vi "adam-4069-basic.vi"() -> ()   [LabVIEW 2024]
uses:
  <vilib>/Instr/_visa.llb/VISA Configure Serial Port (Instr).vi
panel:
  out "Stop Pressed":bool
  out "On Pressed":bool
  out "return count":u32
  out "read buffer":string
  out "error out":errorcluster
  out "return count":u32
  in  "Stop Program":bool
  in  "Off":bool
  in  "On":bool
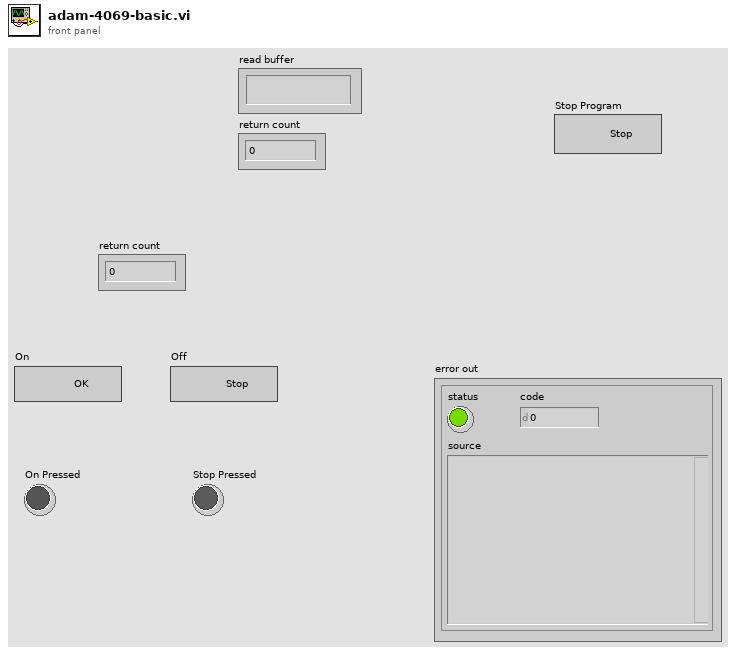
[diagram p1: front panel]
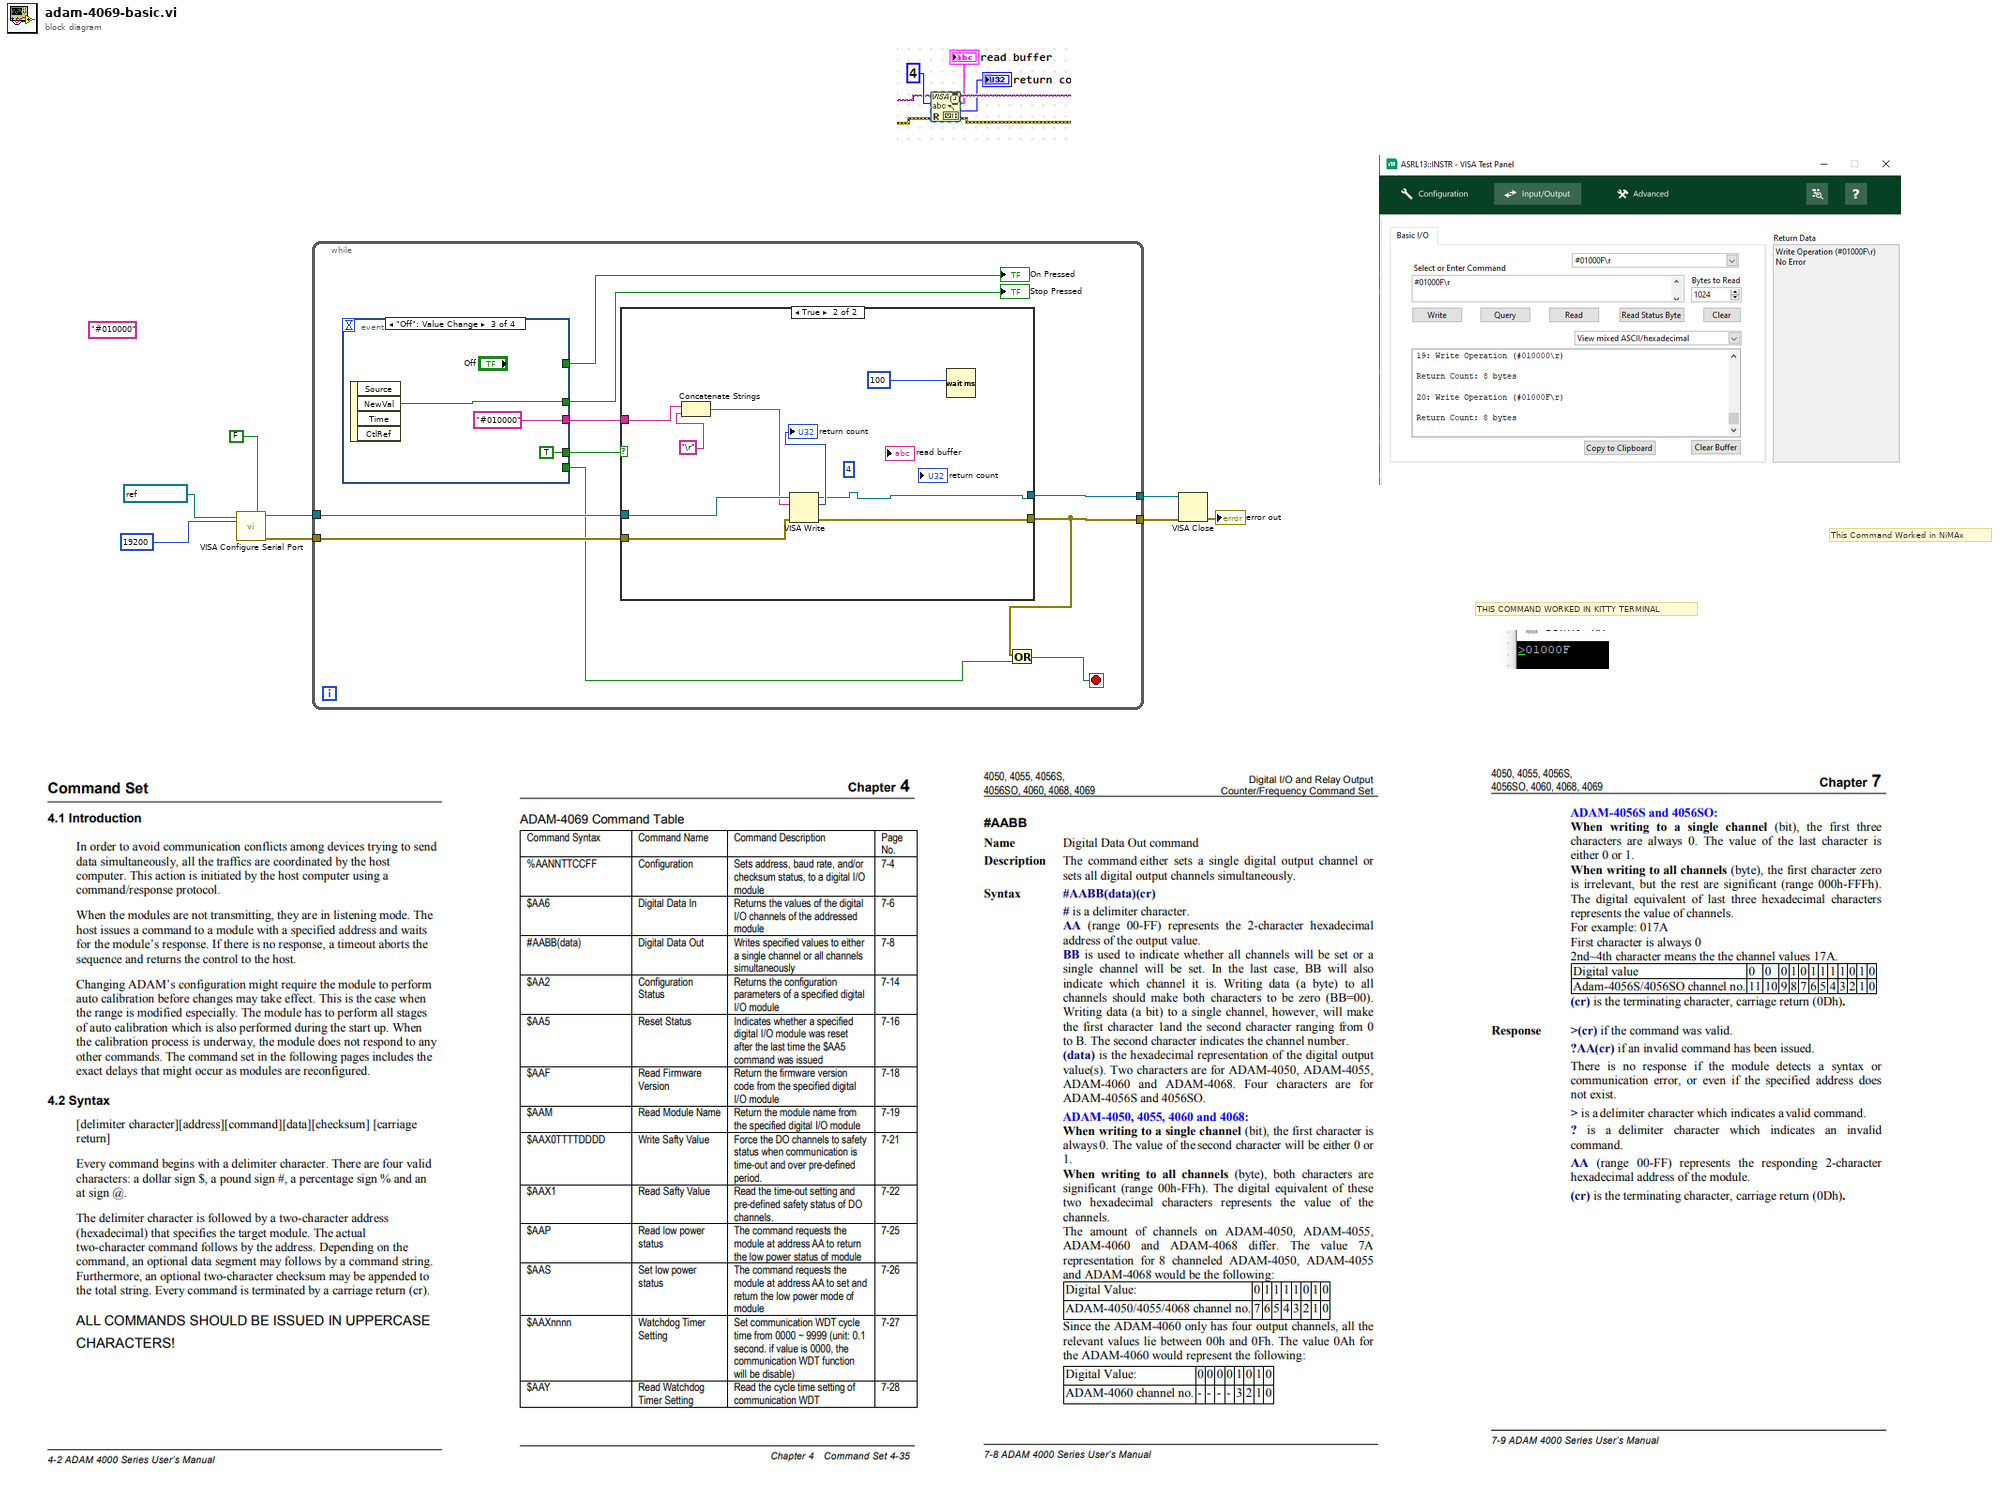
[diagram p0: block diagram]
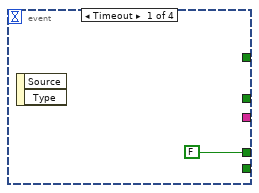
[diagram p2: hidden frame]
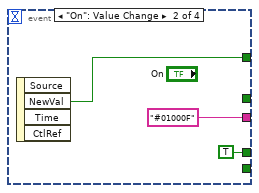
[diagram p3: hidden frame]
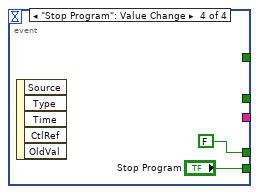
[diagram p4: hidden frame]
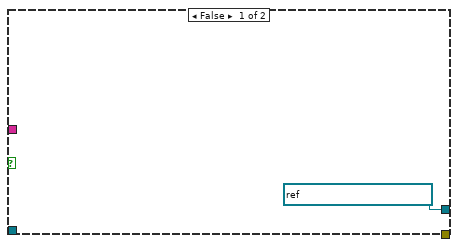
[diagram p5: hidden frame]
diagram:
  (unwired) "#010000" ("write buffer")
  # "This Command Worked in NiMAx"
  # "THIS COMMAND WORKED IN KITTY TERMINAL"
  n1 = call-poly "VISA Configure Serial Port"("VISA resource name"=refnum<visa-resource-name> "COM10", "Enable Termination\nChar (T)"=FALSE ("Enable Termination\nChar (T)"), "baud rate (9600)"=u32 19200) -> ("VISA resource name out"=w3:refnum<visa-resource-name>, "error out"=w2:errorcluster)  [unwired: 11 in]
  n2 = while {
    tunnel: [w18] -> w8
    tunnel: [w9] -> w7
    tunnel: w3 -> [w13]
    tunnel: w2 -> [w12]
    stop <- w10 stop-if-true
    n3 = event shown="[2] \"Off\": Value Change" {
      selector: _ -> [_ _ _ _]
      dyn-events: _ -> [_ _ _ _]
      timeout: _ -> [_ _ _ _]
      tunnel: [_ "#01000F" ("write buffer") "#010000" ("write buffer") _] -> w17
      tunnel: [FALSE TRUE TRUE FALSE] -> w16
      tunnel: [_ _ _ "Stop Program"] -> w11
      tunnel: [_ _ w23 _] -> w15
      tunnel: [_ w20 _ _] -> w14
      event Timeout {
        n4 = event-data() -> ()  [unwired: 1 in, 2 out]
      }
      event "On": Value Change {
        n5 = event-data() -> ("NewVal"=w20:bool)  [unwired: 1 in, 3 out]
      }
      event "Off": Value Change {
        n6 = event-data() -> ("NewVal"=w23:bool)  [unwired: 1 in, 3 out]
      }
      event "Stop Program": Value Change {
        n7 = event-data() -> ()  [unwired: 1 in, 5 out]
      }
    }
    "Stop Pressed" <- w15
    "On Pressed" <- w14
    n8 = case shown="True" w16 {
      tunnel: [refnum<visa-resource-name> "ASRL11::INSTR" ("VISA resource name") w33] -> w18
      tunnel: [_ w32] -> w9
      tunnel: w17 -> [_ w29]
      tunnel: w13 -> [_ w35]
      tunnel: w12 -> [_ w34]
      frame False {
      }
      frame True {
        (unwired) u32 4 ("byte count")
        n9 = Concatenate Strings(w29, "\r") -> (w30:string)
        n10 = VISA Write(VISA resource name=w35, write buffer=w30, error in (no error)=w34) -> (VISA resource name out=w33:refnum<visa-resource-name>, return count=→"return count":u32, error out=w32:errorcluster)
        n11 = Wait (ms)(milliseconds to wait=u32 100) -> ()  [unwired: 1 out]
      }
    }
    n12 = Or(x=w9, y=w11) -> (x .or. y?=w10:bool)
  }
  n13 = VISA Close(VISA resource name=w8, error in (no error)=w7) -> (error out=→"error out":errorcluster)
